vi "Lower stop.vi"(8 "error in (no error)":errorcluster, 9 "Motion.lvclass 2":refnum<class "Motion.lvclass">, 10 "I-O.lvclass":refnum<class "I-O.lvclass">) -> (0 "error out":errorcluster, 1 "Motion.lvclass":refnum<class "Motion.lvclass">, 2 "I-O out":refnum<class "I-O.lvclass">)   [LabVIEW 2016]
uses:
  Classes/Controller/I-O/I-O.lvclass
  Classes/Controller/Motion/Motion.lvclass
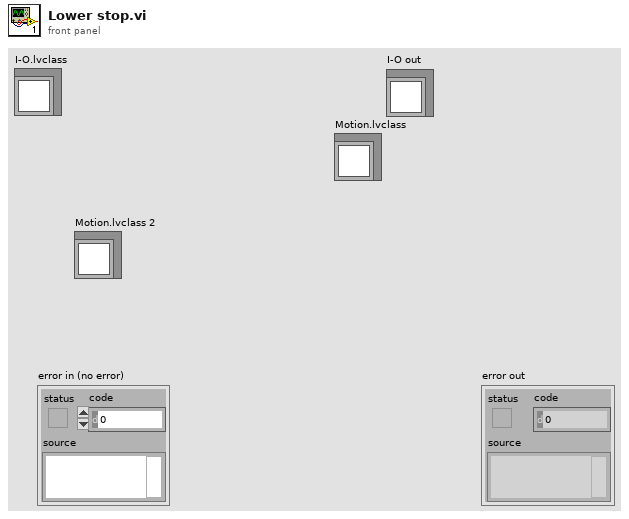
[diagram p1: front panel]
types:
  T1 = typedef "I-O.lvclass/Pin Map.ctl" = cluster{"Region Valves":i32[], "Extra Valves":dbl[][][], "Tool Primary Valve":i32, "Tool Secondary Valve":i32, "Region Sensors":i32[], "Extra Sensors":dbl[][][], "Tool Primary Sensor":dbl, "Tool Secondary Sensor":dbl, "Compression Sensor":dbl, "5V":i32}
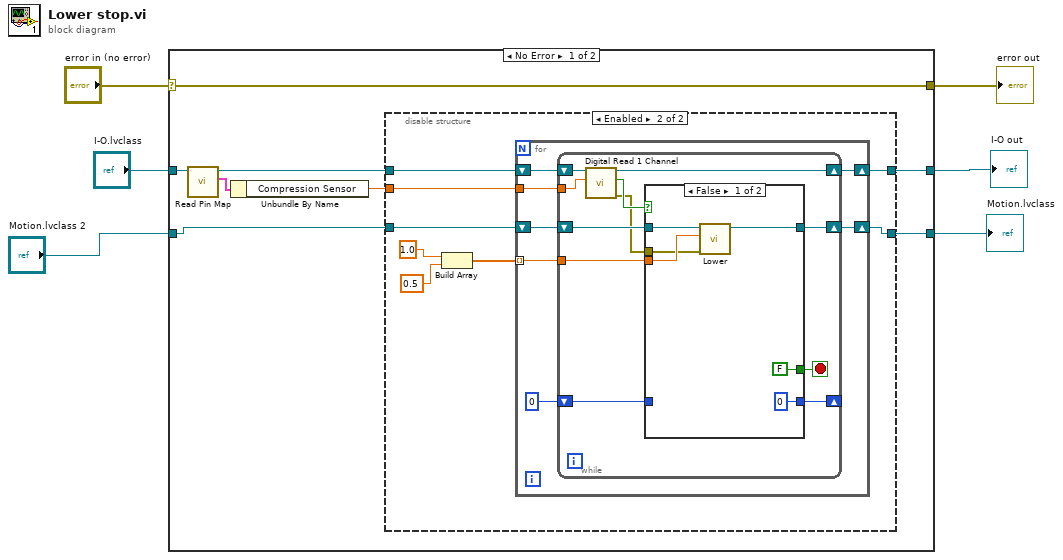
[diagram p0: block diagram]
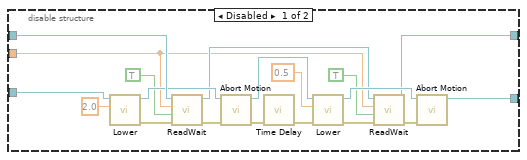
[diagram p2: hidden frame]
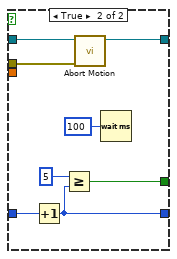
[diagram p3: hidden frame]
diagram:
  n1 = case shown="No Error" "error in (no error)" {
    selector: "error in (no error)" -> [w14 w76]
    tunnel: [w14 w76] -> w5
    tunnel: "I-O.lvclass" -> [w12 w75]
    tunnel: [w7 w75] -> w3
    tunnel: [w8 w74] -> w1
    tunnel: "Motion.lvclass 2" -> [w13 w74]
    frame No Error {
      n2 = call-dynamic "Read Pin Map.vi"("I-O in"=w12) -> ("Pin Map 2"=w10:T1, "I-O out"=w11:refnum<class "I-O.lvclass">)  [unwired: 8 in, 1 out]
      n3 = Unbundle By Name(w10) -> ("Compression Sensor"=w9:dbl)
      n4 = disable-structure shown="Enabled" {
        disable-tunnel: w13 -> [w31 w35]
        disable-tunnel: w11 -> [w30 w40]
        disable-tunnel: w9 -> [w17 w41]
        disable-tunnel: [w16 w34] -> w8
        disable-tunnel: [w15 w39] -> w7
        frame Disabled {
          n5 = call-dynamic "Lower.vi"("Speed"=2.0, "Motion in"=w31) -> ("error out"=w32:errorcluster, "Motion out"=w29:refnum<class "Motion.lvclass">)  [unwired: 8 in]
          n6 = call "ReadWait.vi"("error in (no error)"=w32, "Value"=TRUE, "Read"=w17, "I-O in"=w30) -> ("error out"=w33:errorcluster, "I-O out"=w19:refnum<class "I-O.lvclass">)  [unwired: 6 in]
          n7 = call-dynamic "Abort Motion.vi"("error in (no error)"=w33, "Motion in"=w29) -> ("error out"=w21:errorcluster, "Motion out"=w18:refnum<class "Motion.lvclass">)  [unwired: 8 in]
          n8 = call "Time Delay"("error in (no error)"=w21) -> ("error out"=w20:errorcluster)  [unwired: 10 in]
          n9 = call-dynamic "Lower.vi"("error in (no error)"=w20, "Speed"=0.5, "Motion in"=w18) -> ("error out"=w25:errorcluster, "Motion out"=w24:refnum<class "Motion.lvclass">)  [unwired: 7 in]
          n10 = call "ReadWait.vi"("error in (no error)"=w25, "Value"=TRUE, "Read"=w17, "I-O in"=w19) -> ("error out"=w26:errorcluster, "I-O out"=w15:refnum<class "I-O.lvclass">)  [unwired: 6 in]
          n11 = call-dynamic "Abort Motion.vi"("error in (no error)"=w26, "Motion in"=w24) -> ("Motion out"=w16:refnum<class "Motion.lvclass">)  [unwired: 8 in, 1 out]
        }
        frame Enabled {
          n12 = Build Array(1.0 ("Speed"), 0.5 ("Speed")) -> (w36:dbl[])
          n13 = for {
            tunnel: w41 -> [w48]
            shift-right: [w46] -> w39
            shift-left: w40 -> [w47]
            tunnel: w36 -> [w44] mode=indexing
            shift-right: [w42] -> w34
            shift-left: w35 -> [w43]
            n14 = while {
              tunnel: w48 -> [w59]
              shift-right: [w57] -> w46
              shift-left: w47 -> [w58]
              shift-right: [w53] -> _
              shift-left: 0 -> [w55]
              tunnel: w44 -> [w52]
              shift-right: [w50] -> w42
              shift-left: w43 -> [w51]
              stop <- w54 stop-if-true
              n15 = call-dynamic "Digital Read 1 Channel.vi"("Read"=w59, "I-O in"=w58) -> ("error out"=w49:errorcluster, "Value"=w56:bool, "I-O out"=w57:refnum<class "I-O.lvclass">)  [unwired: 7 in]
              n16 = case shown="False" w56 {
                tunnel: w55 -> [_ w73]
                tunnel: [FALSE w71] -> w54
                tunnel: [0 w70] -> w53
                tunnel: w52 -> [w63 _]
                tunnel: w51 -> [w62 w68]
                tunnel: [w61 w69] -> w50
                tunnel: w49 -> [w60 w67]
                frame False {
                  n17 = call-dynamic "Lower.vi"("error in (no error)"=w60, "Speed"=w63, "Motion in"=w62) -> ("Motion out"=w61:refnum<class "Motion.lvclass">)  [unwired: 7 in, 1 out]
                }
                frame True {
                  n18 = Increment(x=w73) -> (x+1=w70:i32)
                  n19 = Greater Or Equal?(x=5, y=w70) -> (x >= y?=w71:bool)
                  n20 = call-dynamic "Abort Motion.vi"("error in (no error)"=w67, "Motion in"=w68) -> ("Motion out"=w69:refnum<class "Motion.lvclass">)  [unwired: 8 in, 1 out]
                  n21 = Wait (ms)(milliseconds to wait=u32 100) -> ()  [unwired: 1 out]
                }
              }
            }
          }
        }
      }
    }
    frame Error {
    }
  }
  "error out" <- w5
  "I-O out" <- w3
  "Motion.lvclass" <- w1
